vi "CetoniPump_Init.vi"(0 "object in":refnum<class "CetoniPump.lvclass">, 2 "Device Configuration Path":string="C:\\Users\\Public\\Documents\\QmixElements\\Projects\\default_project\\Configurations\\sinle", 5 "error in (no error)":errorcluster) -> (14 "object out":refnum<class "CetoniPump.lvclass">, 19 "error out":errorcluster)   [LabVIEW 2023, in "CetoniPump.lvclass"]
uses:
  CetoniPump.lvclass
  CetoniPump.lvclass/CetoniPump.ctl
  CETONI_SDK/lib/labview/labbCAN_Bus_API/SiUnitPrefix.ctl
  CETONI_SDK/lib/labview/labbCAN_Pump_API/VolumeUnits.ctl
  CETONI_SDK/lib/labview/labbCAN_Bus_API/TimeUnits.ctl
  CETONI_SDK/lib/labview/labbCAN_Bus_API/labbCAN_Bus_API.lvlib
  CETONI_SDK/lib/labview/labbCAN_Pump_API/labbCAN_Pump_API.lvlib
  CETONI_SDK/lib/labview/labbCAN_Valve_API/labbCAN_Valve_API.lvlib
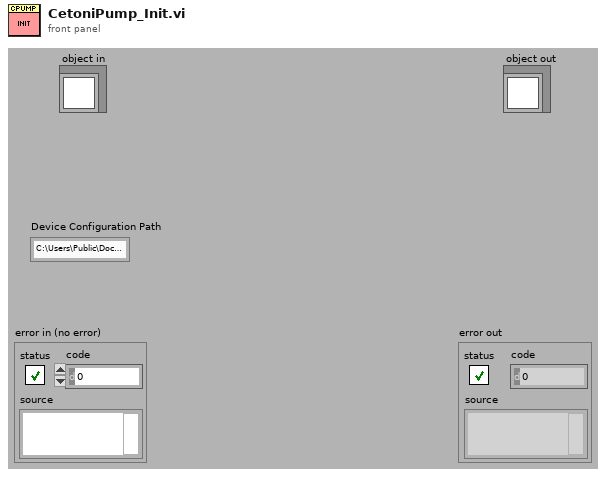
[diagram p1: front panel]
types:
  T1 = cluster{"Pump Handle":i64, "Pump Name":string, "Maximum Volume":dbl, "Maximum Flow Rate":dbl, "Flow Rate":dbl, "Target Level":dbl, "Valve Handle":i64, "Has Valve?":bool, "Actual valve position":i32}[]
  T2 = cluster{"Pump Handle":i64, "Pump Name":string, "Maximum Volume":dbl, "Maximum Flow Rate":dbl, "Flow Rate":dbl, "Target Level":dbl, "Valve Handle":i64, "Has Valve?":bool, "Actual valve position":i32}
  T3 = typedef "labbCAN_Bus_API.lvlib/TimeUnits.ctl" = i32
  T4 = typedef "labbCAN_Pump_API.lvlib/VolumeUnits.ctl" = i32
  T5 = typedef "labbCAN_Bus_API.lvlib/SiUnitPrefix.ctl" = i32
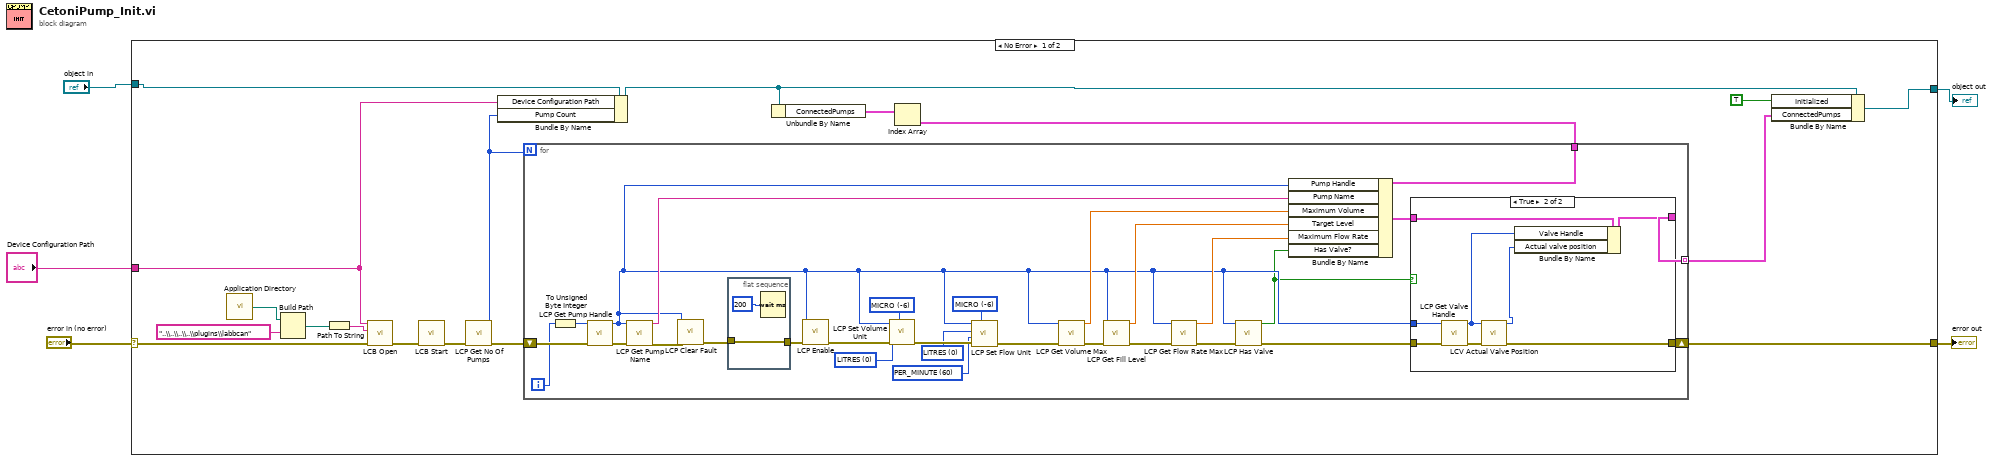
[diagram p0: block diagram]
diagram:
  n1 = case shown="No Error" "error in (no error)" {
    selector: "error in (no error)" -> [w18 w65]
    tunnel: "object in" -> [w23 w66]
    tunnel: [w16 w66] -> w4
    tunnel: [w6 w65] -> w2
    tunnel: "Device Configuration Path" -> [w17 _]
    frame No Error {
      n2 = call <vilib>:"Application Directory.vi"() -> ("Application Directory"=w22:path)
      n3 = Build Path(base path=w22, name or relative path="..\\..\\..\\..\\plugins\\labbcan" ("Name oder relativer Pfad")) -> (appended path=w21:path)
      n4 = Path To String(path=w21) -> (string=w20:string)
      n5 = call "LCB Open.vi"("error in (no error)"=w18, "PluginSearchPath"=w20, "Device Configuration Path"=w17) -> ("error out"=w13:errorcluster)  [unwired: 8 in]
      n6 = call "LCB Start.vi"("error in (no error)"=w13) -> ("error out"=w12:errorcluster)  [unwired: 10 in]
      n7 = call "LCP Get No Of Pumps.vi"("error in (no error)"=w12) -> ("error out"=w14:errorcluster, "Pump Count"=w7:i32)  [unwired: 9 in]
      n8 = Bundle By Name(cluster=w23, "Device Configuration Path"=w17, "Pump Count"=w7) -> (w11:refnum<class "CetoniPump.lvclass">)
      n9 = Unbundle By Name(w11) -> ("ConnectedPumps"=w10:T1)
      n10 = Index Array(array=w10) -> (element=w9:T2)  [unwired: 1 in]
      n11 = for {
        N: w7 -> [_]
        shift-right: [w26] -> w6
        shift-left: w14 -> [w42]
        tunnel: w9 -> [w39]
        tunnel: [w25] -> w8 mode=indexing
        i -> [w32]
        w47 = T3 60 items=["PER_SECOND"=1, "PER_MINUTE"=60, "PER_HOUR"=3600] ("TimeUnit")
        w48 = T4 0 items=["LITRES"] ("VolumeUnit")
        w49 = T4 0 items=["LITRES"] ("Volume Unit")
        w50 = T5 -6 items=["UNIT"=0, "DECI"=-1, "CENTI"=-2, "MILLI"=-3, "MICRO"=-6] ("Prefix")
        w52 = T5 -6 items=["UNIT"=0, "DECI"=-1, "CENTI"=-2, "MILLI"=-3, "MICRO"=-6] ("Prefix")
        n12 = To Unsigned Byte Integer(number=w32) -> (unsigned 8bit integer=w31:u8)
        n13 = call "LCP Get Pump Handle.vi"("error in (no error)"=w42, "Pump Index"=w31) -> ("error out"=w41:errorcluster, "Pump Handle"=w28:i64)  [unwired: 8 in]
        n14 = call "LCP Get Pump Name.vi"("error in (no error)"=w41, "Pump Handle"=w28) -> ("error out"=w40:errorcluster, "Pump Name"=w38:string)  [unwired: 8 in]
        n15 = call "LCP Clear Fault.vi"("error in (no error)"=w40, "Pump Handle"=w28) -> ("error out"=w30:errorcluster)  [unwired: 9 in]
        n16 = flat-sequence {
          tunnel: w30 -> [w63]
          tunnel: [w63] -> w33
          frame #0 {
            n17 = Wait (ms)(milliseconds to wait=u32 200) -> ()  [unwired: 1 out]
          }
        }
        n18 = call "LCP Enable.vi"("error in (no error)"=w33, "Pump Handle"=w28) -> ("error out"=w46:errorcluster)  [unwired: 9 in]
        n19 = call "LCP Set Volume Unit.vi"("Prefix"=w52, "error in (no error)"=w46, "Volume Unit"=w49, "Pump Handle"=w28) -> ("error out"=w51:errorcluster)  [unwired: 7 in]
        n20 = call "LCP Set Flow Unit.vi"("Prefix"=w50, "error in (no error)"=w51, "TimeUnit"=w47, "VolumeUnit"=w48, "Pump Handle"=w28) -> ("error out"=w43:errorcluster)  [unwired: 6 in]
        n21 = call "LCP Get Volume Max.vi"("error in (no error)"=w43, "Pump Handle"=w28) -> ("error out"=w45:errorcluster, "Maximum Volume"=w37:dbl)  [unwired: 8 in]
        n22 = call "LCP Get Fill Level.vi"("error in (no error)"=w45, "Pump Handle"=w28) -> ("error out"=w44:errorcluster, "Fill Level"=w34:dbl)  [unwired: 8 in]
        n23 = call "LCP Get Flow Rate Max.vi"("error in (no error)"=w44, "Pump Handle"=w28) -> ("error out"=w29:errorcluster, "Maximum Flow Rate"=w35:dbl)  [unwired: 8 in]
        n24 = call "LCP Has Valve.vi"("error in (no error)"=w29, "Pump Handle"=w28) -> ("error out"=w27:errorcluster, "Has Valve"=w24:bool)  [unwired: 8 in]
        n25 = Bundle By Name(cluster=w39, "Pump Handle"=w28, "Pump Name"=w38, "Maximum Volume"=w37, "Target Level"=w34, "Maximum Flow Rate"=w35, "Has Valve?"=w24) -> (w36:T2)
        n26 = case shown="True" w24 {
          tunnel: w36 -> [w54 w62]
          tunnel: w28 -> [_ w61]
          tunnel: w27 -> [w53 w60]
          tunnel: [w53 w56] -> w26
          tunnel: [w54 w59] -> w25
          frame False {
          }
          frame True {
            n27 = call "LCP Get Valve Handle.vi"("error in (no error)"=w60, "Pump Handle"=w61) -> ("error out"=w57:errorcluster, "Valve Handle"=w58:i64)  [unwired: 8 in]
            n28 = call "LCV Actual Valve Position.vi"("error in (no error)"=w57, "Valve Handle"=w58) -> ("error out"=w56:errorcluster, "Actual valve position"=w55:i32)  [unwired: 8 in]
            n29 = Bundle By Name(cluster=w62, "Valve Handle"=w58, "Actual valve position"=w55) -> (w59:T2)
          }
        }
      }
      n30 = Bundle By Name(cluster=w11, "Initialized"=TRUE, "ConnectedPumps"=w8) -> (w16:refnum<class "CetoniPump.lvclass">)
    }
    frame Error {
    }
  }
  "object out" <- w4
  "error out" <- w2
